vi "Dashboard USB Camera Loop.vi"(9 "Controller Address":string="10.11.24.11", 10 "Close?":bool, 11 "Refnum in":T1) -> (0 "error out":errorcluster, 2 "Active":bool, 3 "Refnum out":T1, 4 "FPS":dbl, 5 "Bandwidth (Mbps)":dbl)   [LabVIEW 2015]
uses:
  <vilib>/vision/Image Controls.llb/IMAQ Image.ctl
  <vilib>/Rock Robotics/WPI/Camera/WPI_CameraSettings Read MJPG.ctl
  <vilib>/Rock Robotics/WPI/Camera/WPI_CameraImageSize.ctl
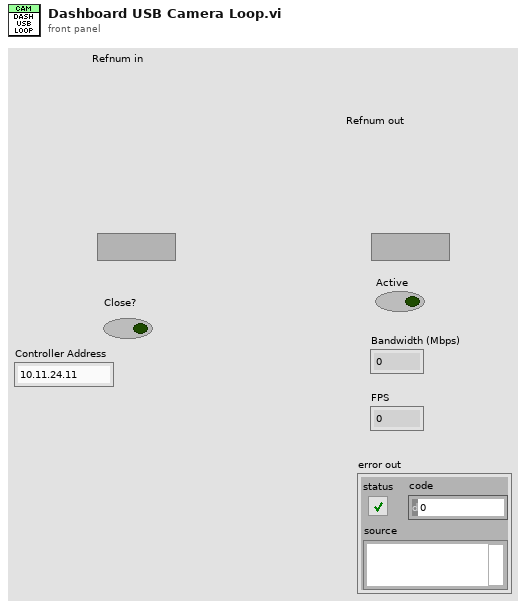
[diagram p1: front panel]
types:
  T1 = typedef "IMAQ Image.ctl" = refnum<image>
  T2 = typedef "WPI_CameraSettings Read MJPG.ctl" = cluster{"fps":i32, "compression":i32, "Image Size":T3}
  T3 = typedef "WPI_CameraImageSize.ctl" = enum16{"640x480", "320x240", "160x120", "Custom"}
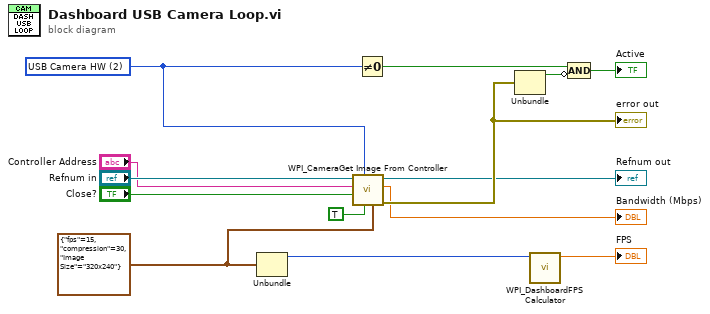
[diagram p0: block diagram]
diagram:
  w8 = T2 {"fps"=15, "compression"=30, "Image Size"=enum."320x240"} ("Camera Settings")
  w4 = u16 2 items=["Camera Off", "USB Camera SW", "USB Camera HW", "IP Camera"] ("Camera Mode")
  n1 = Unbundle(w8) -> ("fps"=w11:i32)  [unwired: 2 out]
  n2 = call <vilib>:"WPI_CameraGet Image From Controller.vi"("Camera Settings"=w8, "USB"=TRUE, "Camera Mode"=w4, "Close?"="Close?", "Controller Address"="Controller Address", "Image"="Refnum in") -> ("error out"=w9:errorcluster, "Bandwidth (Mbps)"=→"Bandwidth (Mbps)":dbl, "Image Out"=→"Refnum out":T1)  [unwired: 3 in]
  "error out" <- w9
  n3 = Not Equal To 0?(x=w4) -> (x != 0?=w10:bool)
  n4 = Unbundle(w9) -> ("status"=w12:bool)  [unwired: 2 out]
  n5 = call <vilib>:"WPI_DashboardFPS Calculator.vi"("Average Count"=w11) -> ("fps"=→"FPS":dbl)  [unwired: 10 in]
  n6 = Compound Arithmetic op=AND(w10, invert w12) -> (→"Active":bool)
